vi "QSBEncoder5.vi"() -> ()   [LabVIEW 2010]
uses:
  C:/Develop/USDigital/QSB/Demos/LabView/QSBLabView2010/USDQSB.dll
  Develop/USDigital/QSB/Demos/LabView/QSBLabView2010/USDQSB.dll
  C:/projects/SIMIS/USDigital/QSBLabView2009/USDQSB.dll
  projects/SIMIS/USDigital/QSBLabView2009/USDQSB.dll
panel:
  in  "Detect Crimp":bool
  out "Waiting For Crimp":bool
  out "Signed Count":i32=1
  out "CrimpTime":u32
  out "CrimpStart":u32
  out "Sampling":bool
  in  "stop":bool
  out "Stopped":bool
  out "Encoder Position":dbl[](array[numeric])=[1.0, 1.0, 1.0, 1.0, 1.0, 1.0, 1.0, 1.0, 1.0, 1.0, 1.0, 1.0, 1.0, 1.0, 1.0, 1.0, 1.0, 1.0, 1.0, 1.0, 1.0, 1.0, 1.0, 1.0, 1.0, 1.0, 1.0, 1.0, 1.0, 1.0, 1.0, 1.0, 1.0, 1.0, 1.0, 1.0, 1.0, 1.0, 1.0, 1.0, 1.0, 1.0, 1.0, 1.0, 1.0, 1.0, 1.0, 1.0, 1.0, 1.0, 1.0, 1.0, 1.0, 1.0, 1.0, 1.0, 1.0, 1.0, 1.0, 1.0, 1.0, 1.0, 1.0, 1.0, 1.0, 1.0, 1.0, 1.0, 1.0, 1.0, 1.0, 1.0, 1.0, 1.0, 1.0, 1.0, 1.0, 1.0, 1.0, 1.0, 1.0, 1.0, 1.0, 1.0, 1.0, 1.0, 1.0, 1.0, 1.0, 1.0, 1.0, 1.0, 1.0, 1.0, 1.0, 1.0, 1.0, 1.0, 1.0, 1.0, 1.0, 1.0, 1.0, 1.0, 1.0, 1.0, 1.0, 1.0, 1.0, 1.0, 1.0, 1.0, 1.0, 1.0, 1.0, 1.0, 1.0, 1.0, 1.0, 1.0, 1.0, 1.0, 1.0, 1.0, 1.0, 1.0, 1.0, 1.0, 1.0, 1.0, 1.0, 1.0, 1.0, 1.0, 1.0, 1.0, 1.0, 1.0, 1.0, 1.0, 1.0, 1.0, 1.0, 1.0, 1.0, 1.0, 1.0, 1.0, 1.0, 1.0, 1.0, 1.0, 1.0, 1.0, 1.0, 1.0, 1.0, 1.0, 1.0, 1.0, 1.0, 1.0, 1.0, 1.0, 1.0, 1.0, 1.0, 1.0, 1.0, 1.0, 1.0, 1.0, 1.0, 1.0, 1.0, 1.0, 1.0, 1.0, 1.0, 1.0, 1.0, 1.0, 1.0, 1.0, 0.0, 0.0, 0.0, 0.0, 0.0, 0.0, 0.0, 0.0, 0.0, 0.0, 0.0, 0.0, 0.0, 0.0, 0.0, 0.0, 0.0, 0.0, 0.0, 0.0, 0.0, 0.0, 0.0, 0.0, 0.0, 0.0, 0.0, 0.0, 0.0, 0.0, 0.0, 0.0, 0.0, 0.0, 0.0, 0.0, 0.0, 0.0, 0.0, 0.0, 0.0, 0.0, 0.0, 0.0, 0.0, 0.0, 0.0, 0.0, 0.0, 0.0, 0.0, 0.0, 0.0, 0.0, 0.0, 0.0, 0.0, 0.0, 0.0, 0.0, 0.0, 0.0, 0.0, 0.0, 0.0, 0.0, 0.0, 0.0, 0.0, 0.0, 0.0, 0.0, 0.0, 0.0, 0.0, 0.0, 0.0, 0.0, 0.0, 0.0, 0.0, 0.0, 0.0, 0.0, 0.0, 0.0, 0.0, 0.0, 0.0, 0.0, 0.0, 0.0, 0.0, 0.0, 0.0, 0.0, 0.0, 0.0, 0.0, 0.0, 0.0, 0.0, 0.0, 0.0, 0.0, 0.0, 0.0, 0.0, 0.0, 0.0, 0.0, 0.0, 1.0, 1.0, 1.0, 1.0, 1.0, 1.0, 1.0, 1.0, 1.0, 1.0, 1.0, 1.0, 1.0, 1.0, 1.0, 1.0, 1.0, 1.0, 1.0, 1.0, 1.0, 1.0, 1.0, 1.0, 1.0, 1.0, 1.0, 1.0, 1.0, 1.0, 1.0, 1.0, 1.0, 1.0, 1.0, 1.0, 1.0, 1.0, 1.0, 1.0, 1.0, 1.0, 1.0, 1.0, 1.0, 1.0, 1.0, 1.0, 1.0, 1.0, 1.0, 1.0, 1.0, 1.0, 1.0, 1.0, 1.0, 1.0, 1.0, 1.0, 1.0, 1.0, 1.0, 1.0, 1.0, 1.0, 1.0, 1.0, 1.0, 1.0, 1.0, 1.0, 1.0, 1.0, 1.0, 1.0, 1.0, 1.0, 1.0, 1.0, 1.0, 1.0, 1.0, 1.0, 1.0, 1.0, 1.0, 1.0, 1.0, 1.0, 1.0, 1.0, 1.0, 1.0, 1.0, 1.0, 1.0, 1.0, 1.0, 1.0, 1.0, 1.0, 1.0, 1.0, 1.0, 1.0, 1.0, 1.0, 1.0, 1.0, 1.0, 1.0, 1.0, 1.0, 1.0, 1.0, 1.0, 1.0, 1.0, 1.0, 1.0, 1.0, 1.0, 1.0, 1.0, 1.0, 1.0, 1.0, 1.0, 1.0, 1.0, 1.0, 1.0, 1.0, 1.0, 1.0, 1.0, 1.0, 1.0, 1.0, 1.0, 1.0, 1.0, 1.0, 1.0, 1.0, 1.0, 1.0, 1.0, 1.0, 1.0, 1.0, 1.0, 1.0, 1.0, 1.0, 1.0, 1.0, 1.0, 1.0, 1.0, 1.0, 1.0, 1.0, 1.0, 1.0, 1.0, 1.0, 1.0, 1.0, 1.0, 1.0, 1.0, 1.0, 1.0, 1.0, 1.0, 1.0, 1.0, 1.0, 1.0, 1.0, 1.0, 1.0, 1.0, 1.0, 1.0, 1.0, 1.0, 1.0, 1.0, 1.0, 1.0, 1.0, 1.0, 1.0, 1.0, 1.0, 1.0, 1.0, 1.0, 1.0, 1.0, 1.0] format="%.2f"
  out "waveform output (graph)":waveform(dbl)(graph)
  in  "Range":dbl=40000.0
  out "Current Position":dbl=1.0
  out "Encoder Count":i32(slide)=1 scale=-30000.0..40000.0
  out "Minimum (msec)":u32=4294967295
  out "Maximum (msec)":u32
  out "Numeric":i32
  out "Connected":bool
  in  "Port Name i.e. COM3":string="COM3"
  out "Connection Status":string="Not Connected"
  in  "Connect":bool
  in  "OFF":bool caption="ON"
  out "Invert Direction":bool
  in  "OFF":bool=TRUE caption="ON"
  out "Enable Counter":bool=TRUE
  out "Sign Bit Set":bool=TRUE
  out "Count Increase":bool
  out "Counter Enabled":bool=TRUE
  out "Index":bool=TRUE
  out "Match":bool
  out "Rollunder":bool=TRUE
  out "Rollover":bool=TRUE
  out "Status (hex)":u32=217 format="%x"
  in  "Clear Status":bool caption="Clear"
  in  "OFF":bool caption="ON"
  out "Trigger On Index":bool
  in  "OFF":bool caption="ON"
  in  "OFF":bool caption="ON"
  out "Trigger On Match":bool
  out "Trigger On Rollunder":bool
  in  "OFF":bool caption="ON"
  out "Trigger On Rollover":bool
  in  "Index Configuration":T1(ring)=enum."Reset Counter"
  out "Index Configuration":string="Reset Counter"
  in  "Counter Mode":T2(ring)
  in  "Reset Count":bool caption="Reset"
  out "Resolution":i32=60001
  out "Counter Mode":string="Free Running"
  out "Quadrature Mode":string="X4"
  in  "Quadrature Mode":enum16{"Clock and Direction", "X1", "X2", "X4"}(ring)=enum."X4"
  in  "Apply":bool
  out "error out":errorcluster
  in  "Input Resolution":i32=60001 max=131071 step=100
  in  "error in (no error)":errorcluster
  # "Encoder Configuration"
  # "Encoder Status"
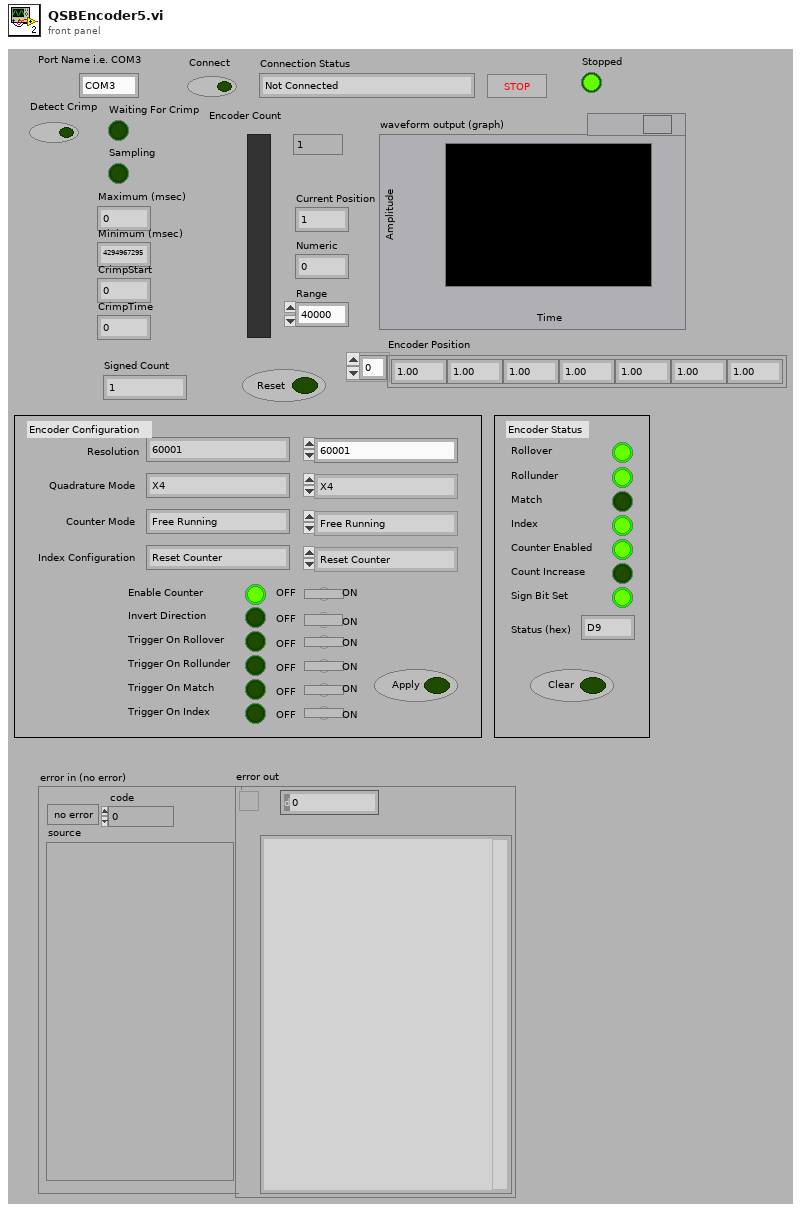
[diagram p1: front panel]
types:
  T1 = enum16{"Disabled", "Preset Counter", "Reset Counter", "Capture Counter"}
  T2 = enum16{"Free Running", "Non-Recycle", "Range Limit", "Modulo-N"}
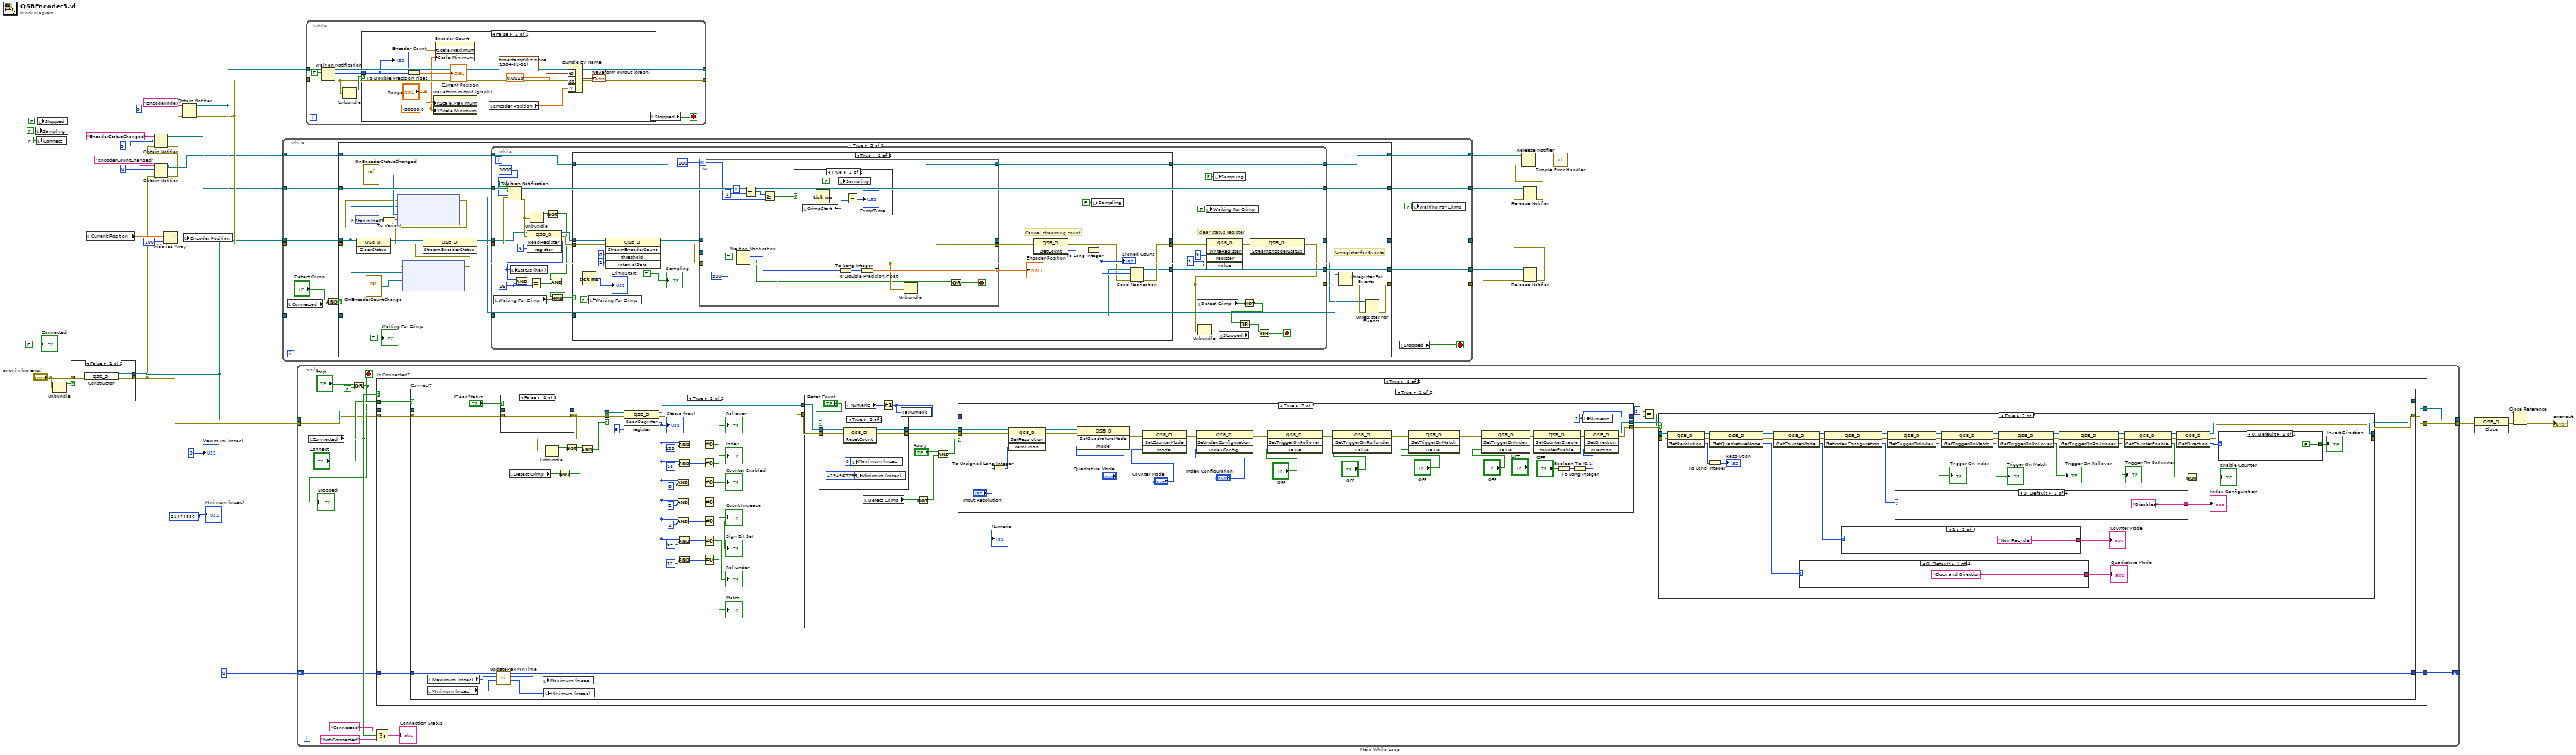
[diagram p0: block diagram]
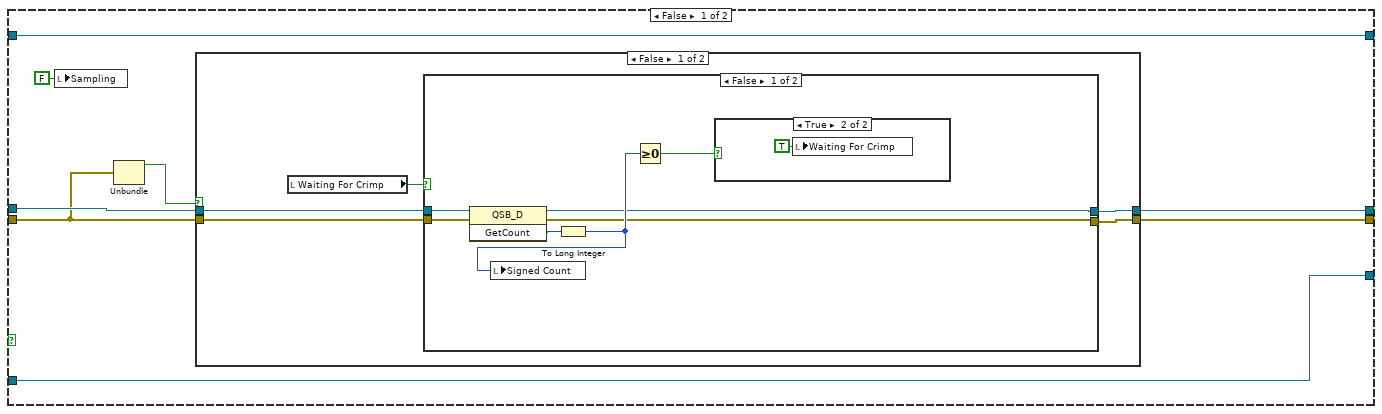
[diagram p4: hidden frame]
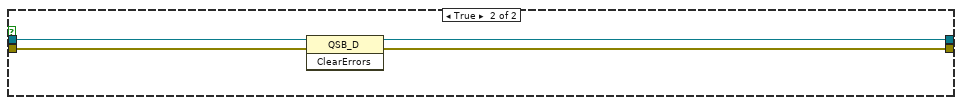
[diagram p7: hidden frame]
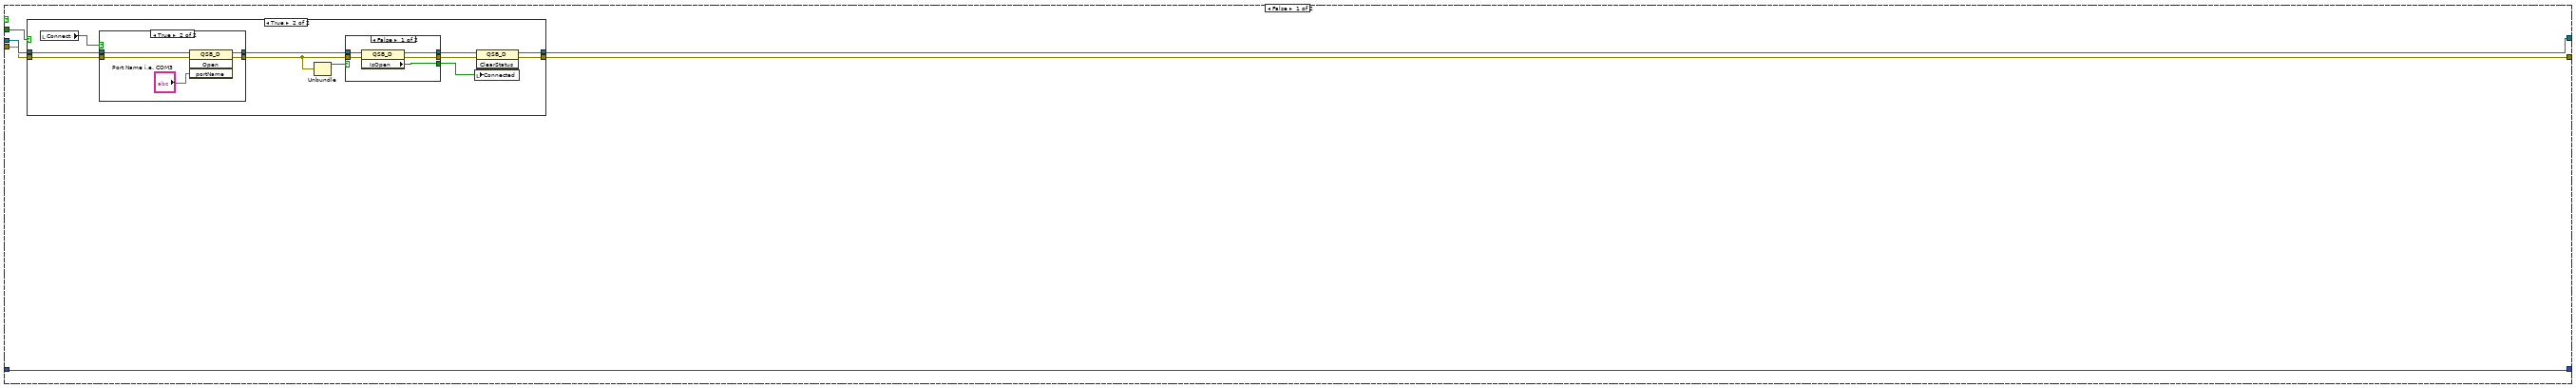
[diagram p9: hidden frame]
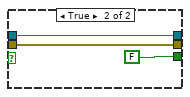
[diagram p11: hidden frame]
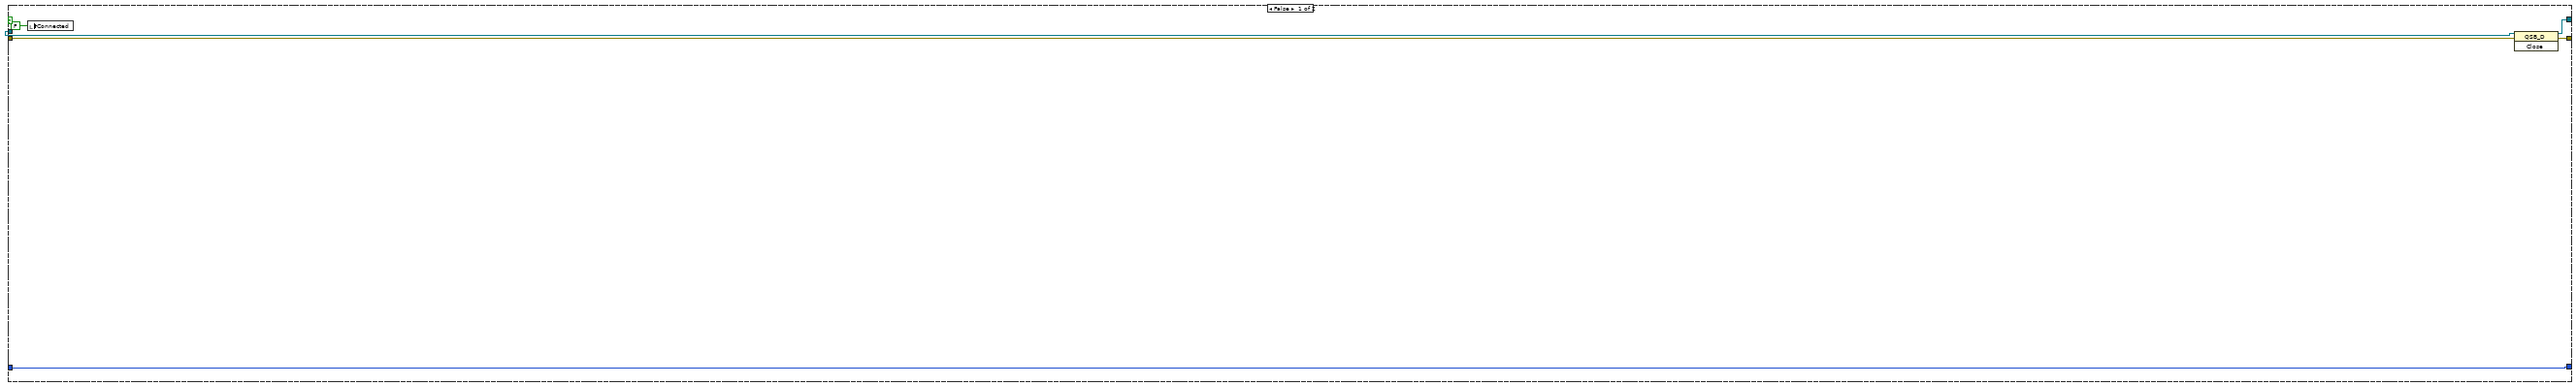
[diagram p13: hidden frame]
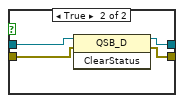
[diagram p15: hidden frame]
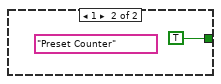
[diagram p18: hidden frame]
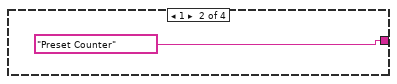
[diagram p19: hidden frame]
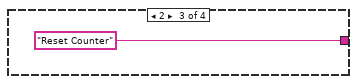
[diagram p20: hidden frame]
diagram:
  n1 = local write "Sampling"(FALSE ("Sampling")) -> ()
  n2 = local write "Connect"(FALSE ("Connect")) -> ()
  n3 = local write "Stopped"(FALSE ("Stopped")) -> ()
  n4 = Unbundle("error in (no error)") -> ("status"=w38:bool)  [unwired: 2 out]
  n5 = case shown="False" w38 {
    tunnel: [w39 refnum<k24> refnum ("new reference")] -> w12
    tunnel: "error in (no error)" -> [w41 w43]
    tunnel: [w40 w43] -> w6
    frame False {
      n6 = constructor class="QSB_D"(error in=w41) -> (reference out=w39:refnum<k24>, error out=w40:errorcluster)  [unwired: 2 in, 1 out]
    }
    frame True {
    }
  }
  n7 = local read "Current Position"() -> (w26:dbl)
  n8 = Obtain Notifier(name (unnamed)="EncoderCountChanged", notification data type=0, error in (no error)=w6) -> (notifier out=w4:refnum<notifier>, error out=w5:errorcluster)  [unwired: 1 in, 1 out]
  n9 = Obtain Notifier(name (unnamed)="EncoderStatusChanged", notification data type=u32 0, error in (no error)=w5) -> (notifier out=w15:refnum<notifier>, error out=w9:errorcluster)  [unwired: 1 in, 1 out]
  n10 = Initialize Array(w26, 100 ("dimension size")) -> (w10:dbl[])
  n11 = Obtain Notifier(name (unnamed)="EncoderIndex", notification data type=0, error in (no error)=w9) -> (notifier out=w24:refnum<notifier>, error out=w23:errorcluster)  [unwired: 1 in, 1 out]
  n12 = local write "Encoder Position"(w10) -> ()
  n13 = while {
    tunnel: w12 -> [w54]
    tunnel: w23 -> [w53]
    tunnel: w24 -> [w58]
    tunnel: [w57] -> w28
    tunnel: [w56] -> w11
    tunnel: w15 -> [w49]
    tunnel: [w47] -> w14
    tunnel: [w46] -> _
    tunnel: w4 -> [w45]
    tunnel: [w44] -> w1
    stop <- w55 stop-if-true
    n14 = local read "Connected"() -> (w51:bool)
    n15 = And(x="Detect Crimp", y=w51) -> (x .and. y?=w52:bool)
    n16 = case shown="True" w52 {
      tunnel: w54 -> [w60 w70]
      tunnel: w53 -> [w63 w76]
      tunnel: w58 -> [w62 w88]
      tunnel: [w62 w87] -> w57
      tunnel: [w63 w66] -> w56
      tunnel: w49 -> [w61 w85]
      tunnel: [w61 w84] -> w47
      tunnel: [w60 w74] -> w46
      tunnel: w45 -> [w59 w73]
      tunnel: [w59 w72] -> w44
      frame False {
      }
      frame True {
        # "Unregister for Events"
        n17 = control-ref of="Status (hex)"() -> (w82:refnum<vi>)
        n18 = invoke class="QSB_D" method="ClearStatus"(reference=w70, error in=w76) -> (reference out=w77:refnum<k24>, error out=w75:errorcluster)  [unwired: 1 in, 1 out]
        n19 = vi-ref <userlib>:"OnEncoderStatusChanged.vi"() -> ("vi reference"=w79:refnum<vi>)
        n20 = vi-ref <userlib>:"OnEncoderCountChange.vi"() -> ("vi reference"=w71:refnum<vi>)
        n21 = To Variant(anything=w82) -> (Variant=w83:variant)
        n22 = node(w75, w70, w79, w83) -> (w65:refnum<k27>, w69:errorcluster)  [unwired: 1 in]
        n23 = node(w69, w70, w71) -> (w64:refnum<k27>, w68:errorcluster)  [unwired: 2 in]
        n24 = invoke class="QSB_D" method="StreamEncoderStatus"(reference=w77, error in=w68) -> (reference out=w81:refnum<k24>, error out=w80:errorcluster)  [unwired: 1 in, 1 out]
        n25 = while {
          tunnel: w80 -> [w118]
          tunnel: w88 -> [w125]
          tunnel: w81 -> [w105]
          tunnel: [w124] -> w87
          tunnel: [w109] -> w78
          tunnel: w85 -> [w119]
          tunnel: [w113] -> w84
          tunnel: [w108] -> w74
          tunnel: w73 -> [w92]
          tunnel: [w91] -> w72
          stop <- w123 stop-if-true
          w126 = u32 16 ("y")
          # "clear status register"
          n26 = local read "Waiting For Crimp"() -> (w96:bool)
          n27 = Wait on Notification(notifier=w119, ignore previous (F)=TRUE, timeout in ms (-1)=1000, error in (no error)=w118) -> (notifier out=w113:refnum<notifier>, error out=w107:errorcluster)  [unwired: 2 out]
          n28 = invoke class="QSB_D" method="ReadRegister"(reference=w105, error in=w107, "register"=u8 6) -> (reference out=w104:refnum<k24>, error out=w106:errorcluster, "ReadRegister"=w94:u32)  [unwired: 1 in, 1 out]
          n29 = local write "Status (hex)"(w94) -> ()
          n30 = And(x=w94, y=w126) -> (x .and. y?=w127:u32)
          n31 = Equal?(x=w127, y=w126) -> (x = y?=w116:bool)
          n32 = Unbundle(w107) -> ("status"=w117:bool)  [unwired: 2 out]
          n33 = Not(x=w117) -> (.not. x?=w95:bool)
          n34 = And(x=w95, y=w116) -> (x .and. y?=w111:bool)
          n35 = And(x=w111, y=w96) -> (x .and. y?=w110:bool)
          n36 = case shown="True" w110 {
            tunnel: w106 -> [w130 w156]
            tunnel: w125 -> [w135 w173]
            tunnel: [w135 w175] -> w124
            tunnel: [w131 w176] -> w99
            tunnel: w104 -> [w133 w163]
            tunnel: [w132 w161] -> w100
            tunnel: w92 -> [w128 w157]
            tunnel: [w128 w159] -> w91
            frame False {
              n37 = local write "Sampling"(FALSE ("Sampling")) -> ()
              n38 = Unbundle(w130) -> ("status"=w129:bool)  [unwired: 2 out]
              n39 = case shown="False" w129 {
                tunnel: w133 -> [w139 w154]
                tunnel: [w138 w152] -> w132
                tunnel: w130 -> [w137 w153]
                tunnel: [w136 w151] -> w131
                frame False {
                  n40 = local read "Waiting For Crimp"() -> (w140:bool)
                  n41 = case shown="False" w140 {
                    tunnel: w139 -> [w147 w150]
                    tunnel: [w142 w150] -> w138
                    tunnel: w137 -> [w146 w149]
                    tunnel: [w141 w149] -> w136
                    frame False {
                      n42 = invoke class="QSB_D" method="GetCount"(reference=w147, error in=w146) -> (reference out=w142:refnum<k24>, error out=w141:errorcluster, "GetCount"=w145:u32)  [unwired: 1 in]
                      n43 = To Long Integer(number=w145) -> (32bit integer=w144:i32)
                      n44 = local write "Signed Count"(w144) -> ()
                      n45 = Greater Or Equal To 0?(x=w144) -> (x >= 0?=w143:bool)
                      n46 = case shown="True" w143 {
                        frame False {
                        }
                        frame True {
                          n47 = local write "Waiting For Crimp"(TRUE ("Waiting For Crimp")) -> ()
                        }
                      }
                    }
                    frame True {
                    }
                  }
                }
                frame True {
                  n48 = invoke class="QSB_D" method="ClearErrors"(reference=w154, error in=w153) -> (reference out=w152:refnum<k24>, error out=w151:errorcluster)  [unwired: 1 in, 1 out]
                }
              }
            }
            frame True {
              # "Cancel streaming count"
              n49 = Tick Count (ms)() -> (millisecond timer value=→"CrimpStart":u32)
              n50 = local write "Waiting For Crimp"(FALSE ("Waiting For Crimp")) -> ()
              n51 = invoke class="QSB_D" method="StreamEncoderCount"(reference=w163, error in=w156, "threshold"=u32 0, "intervalRate"=u32 1) -> (reference out=w165:refnum<k24>, error out=w167:errorcluster)  [unwired: 1 in, 3 out]
              n52 = for {
                N: 100 -> [w190]
                tunnel: [w194] -> w170 mode=indexing
                tunnel: [w184] -> w158
                tunnel: w167 -> [w185]
                tunnel: w165 -> [w186]
                tunnel: [w186] -> w162
                tunnel: w157 -> [w188]
                tunnel: [w187] -> w159
                i -> [w189]
                stop <- w179 stop-if-true
                n53 = Wait on Notification(notifier=w188, ignore previous (F)=TRUE, timeout in ms (-1)=500, error in (no error)=w185) -> (notifier out=w187:refnum<notifier>, notification=w183:i32, timed out?=w178:bool, error out=w184:errorcluster)
                n54 = Add(x=w189, y=1) -> (x+y=w191:i32)
                n55 = Greater Or Equal?(x=w191, y=w190) -> (x >= y?=w192:bool)
                n56 = case shown="True" w192 {
                  frame False {
                  }
                  frame True {
                    n57 = local read "CrimpStart"() -> (w199:u32)
                    n58 = Tick Count (ms)() -> (millisecond timer value=w198:u32)
                    n59 = local write "Sampling"(FALSE ("Sampling")) -> ()
                    n60 = Subtract(x=w198, y=w199) -> (x-y=→"CrimpTime":u32)
                  }
                }
                n61 = To Long Integer(number=w183) -> (32bit integer=w195:i32)
                n62 = To Double Precision Float(number=w195) -> (double precision float=w194:dbl)
                n63 = Unbundle(w184) -> ("status"=w180:bool)  [unwired: 2 out]
                n64 = Or(x=w178, y=w180) -> (x .or. y?=w179:bool)
              }
              "Encoder Position" <- w170
              n65 = invoke class="QSB_D" method="GetCount"(reference=w162, error in=w158) -> (reference out=w161:refnum<k24>, error out=w155:errorcluster, "GetCount"=w160:u32)  [unwired: 1 in]
              n66 = To Long Integer(number=w160) -> (32bit integer=w174:i32)
              "Signed Count" <- w174
              n67 = local write "Sampling"(FALSE ("Sampling")) -> ()
              n68 = Send Notification(notification=w174, notifier=w173, error in (no error)=w155) -> (notifier out=w175:refnum<notifier>, error out=w176:errorcluster)
              "Sampling" <- TRUE ("Sampling")
            }
          }
          n69 = local read "Detect Crimp"() -> (w115:bool)
          n70 = local write "Waiting For Crimp"(TRUE ("Waiting For Crimp")) -> ()
          n71 = invoke class="QSB_D" method="WriteRegister"(reference=w100, error in=w99, "register"=u8 9, "value"=u32 3) -> (reference out=w98:refnum<k24>, error out=w97:errorcluster)  [unwired: 1 in, 3 out]
          n72 = local write "Sampling"(FALSE ("Sampling")) -> ()
          n73 = local read "Stopped"() -> (w120:bool)
          n74 = Not(x=w115) -> (.not. x?=w90:bool)
          n75 = invoke class="QSB_D" method="StreamEncoderStatus"(reference=w98, error in=w97) -> (reference out=w108:refnum<k24>, error out=w109:errorcluster)  [unwired: 1 in, 1 out]
          n76 = Unbundle(w109) -> ("status"=w121:bool)  [unwired: 2 out]
          n77 = Or(x=w90, y=w121) -> (x .or. y?=w122:bool)
          n78 = Or(x=w122, y=w120) -> (x .or. y?=w123:bool)
        }
        n79 = Unregister For Events(event registration refnum=w65, error in=w78) -> (error out=w67:errorcluster)
        n80 = Unregister For Events(event registration refnum=w64, error in=w67) -> (error out=w66:errorcluster)
        "Waiting For Crimp" <- TRUE ("Waiting For Crimp")
      }
    }
    n81 = local read "Stopped"() -> (w55:bool)
    n82 = local write "Waiting For Crimp"(FALSE ("Waiting for Crimp")) -> ()
  }
  n83 = while "Main While Loop" {
    tunnel: [w213] -> w33
    tunnel: [w212] -> w32
    tunnel: w12 -> [w206]
    tunnel: w6 -> [w205]
    shift-right: [w202] -> _
    shift-left: u32 0 -> [w203]
    stop <- w200 stop-if-true
    n84 = local read "Connected"() -> (w209:bool)
    n85 = Or(x="stop", y=FALSE) -> (x .or. y?=w200:bool)
    "Stopped" <- w200
    n86 = Select(t="Connected", s=w209, f="Not Connected") -> (s? t:f=→"Connection Status":string)
    n87 = case "Is Connected?" shown="True" w209 {
      tunnel: [w216 w254] -> w213
      tunnel: [w215 w253] -> w212
      tunnel: "Connect" -> [w219 w252]
      tunnel: w206 -> [w218 w250]
      tunnel: w205 -> [w217 w251]
      tunnel: w203 -> [w214 w249]
      tunnel: [w214 w248] -> w202
      frame False {
        n88 = case shown="True" w219 {
          tunnel: w218 -> [w220 w229]
          tunnel: w217 -> [w221 w228]
          tunnel: [w221 w223] -> w215
          tunnel: [w220 w222] -> w216
          frame False {
          }
          frame True {
            n89 = local read "Connect"() -> (w226:bool)
            n90 = case shown="True" w226 {
              tunnel: [w242 w247] -> w231
              tunnel: [w241 w246] -> w230
              tunnel: w229 -> [w242 w244]
              tunnel: w228 -> [w241 w243]
              frame False {
              }
              frame True {
                n91 = invoke on="Invoke Node" class="QSB_D" method="Open"(reference=w244, error in=w243, "portName"="Port Name i.e. COM3") -> (reference out=w247:refnum<k24>, error out=w246:errorcluster)  [unwired: 1 in, 2 out]
              }
            }
            n92 = Unbundle(w230) -> ("status"=w232:bool)  [unwired: 2 out]
            n93 = case shown="False" w232 {
              tunnel: [w237 w239] -> w224
              tunnel: [w236 w240] -> w225
              tunnel: w231 -> [w234 w239]
              tunnel: w230 -> [w235 w240]
              tunnel: [w233 FALSE] -> w227
              frame False {
                n94 = property class="QSB_D"(reference=w234, error in=w235) -> (reference out=w237:refnum<k24>, error out=w236:errorcluster, "IsOpen"=w233:bool)
              }
              frame True {
              }
            }
            n95 = local write "Connected"(w227) -> ()
            n96 = invoke class="QSB_D" method="ClearStatus"(reference=w224, error in=w225) -> (reference out=w222:refnum<k24>, error out=w223:errorcluster)  [unwired: 1 in, 1 out]
          }
        }
      }
      frame True {
        n97 = case "Connect?" shown="True" w252 {
          tunnel: [w257 w292] -> w254
          tunnel: [w258 w291] -> w253
          tunnel: w251 -> [w260 w277]
          tunnel: w250 -> [w259 w276]
          tunnel: w249 -> [w255 w272]
          tunnel: [w255 w271] -> w248
          frame False {
            n98 = local write "Connected"(FALSE) -> ()
            n99 = invoke class="QSB_D" method="Close"(reference=w259, error in=w260) -> (reference out=w257:refnum<k24>, error out=w258:errorcluster)  [unwired: 1 in, 1 out]
          }
          frame True {
            n100 = local read "Minimum (msec)"() -> (w269:u32)
            n101 = local read "Maximum (msec)"() -> (w270:u32)
            n102 = call <userlib>:"UpdateMaxMinTime.vi"("Minimum (msec)"=w269, "Maximum (msec)"=w270, "LastTime (msec)"=w272) -> ("MinimumOut (msec)"=w267:u32, "MaximumOut (msec)"=w268:u32, "LastTimeOut (msec)"=w271:u32)  [unwired: 6 in]
            n103 = case shown="False" "Clear Status" {
              tunnel: [w303 w307] -> w287
              tunnel: [w304 w305] -> w286
              tunnel: w276 -> [w303 w308]
              tunnel: w277 -> [w304 w306]
              frame False {
              }
              frame True {
                n104 = invoke class="QSB_D" method="ClearStatus"(reference=w308, error in=w306) -> (reference out=w307:refnum<k24>, error out=w305:errorcluster)  [unwired: 1 in, 1 out]
              }
            }
            n105 = local read "Detect Crimp"() -> (w275:bool)
            n106 = local write "Maximum (msec)"(w268) -> ()
            n107 = local write "Minimum (msec)"(w267) -> ()
            n108 = Unbundle(w286) -> ("status"=w265:bool)  [unwired: 2 out]
            n109 = Not(x=w275) -> (.not. x?=w274:bool)
            n110 = Not(x=w265) -> (.not. x?=w266:bool)
            n111 = And(x=w266, y=w274) -> (x .and. y?=w273:bool)
            n112 = case shown="True" w273 {
              tunnel: w286 -> [w310 w337]
              tunnel: w287 -> [w309 w336]
              tunnel: [w309 w335] -> w284
              tunnel: [w310 w333] -> w285
              frame False {
              }
              frame True {
                n113 = invoke on="Invoke Node" class="QSB_D" method="ReadRegister"(reference=w336, error in=w337, "register"=6) -> (reference out=w335:refnum<k24>, error out=w333:errorcluster, "ReadRegister"=w311:u32)  [unwired: 1 in, 1 out]
                "Status (hex)" <- w311
                n114 = And(x=w311, y=8) -> (x .and. y?=w319:u32)
                n115 = And(x=w311, y=2) -> (x .and. y?=w316:u32)
                n116 = And(x=w311, y=1) -> (x .and. y?=w313:u32)
                n117 = And(x=w311, y=128) -> (x .and. y?=w331:u32)
                n118 = And(x=w311, y=16) -> (x .and. y?=w322:u32)
                n119 = And(x=w311, y=64) -> (x .and. y?=w328:u32)
                n120 = And(x=w311, y=32) -> (x .and. y?=w325:u32)
                n121 = Not Equal To 0?(x=w331) -> (x != 0?=→"Rollover":bool)
                n122 = Not Equal To 0?(x=w322) -> (x != 0?=→"Index":bool)
                n123 = Not Equal To 0?(x=w319) -> (x != 0?=→"Counter Enabled":bool)
                n124 = Not Equal To 0?(x=w316) -> (x != 0?=→"Count Increase":bool)
                n125 = Not Equal To 0?(x=w313) -> (x != 0?=→"Sign Bit Set":bool)
                n126 = Not Equal To 0?(x=w328) -> (x != 0?=→"Rollunder":bool)
                n127 = Not Equal To 0?(x=w325) -> (x != 0?=→"Match":bool)
              }
            }
            n128 = case shown="True" "Reset Count" {
              tunnel: w285 -> [w295 w302]
              tunnel: w284 -> [w296 w301]
              tunnel: [w296 w300] -> w283
              tunnel: [w295 w299] -> w282
              frame False {
              }
              frame True {
                n129 = invoke class="QSB_D" method="ResetCount"(reference=w301, error in=w302) -> (reference out=w300:refnum<k24>, error out=w299:errorcluster)  [unwired: 1 in, 1 out]
                n130 = local write "Maximum (msec)"(u32 0 ("Maximum (msec)")) -> ()
                n131 = local write "Minimum (msec)"(u32 4294967295 ("Minimum (msec)")) -> ()
              }
            }
            n132 = local read "Numeric"() -> (w290:i32)
            n133 = local read "Detect Crimp"() -> (w262:bool)
            n134 = Increment(x=w290) -> (x+1=w289:i32)
            n135 = local write "Numeric"(w289) -> ()
            n136 = Not(x=w262) -> (.not. x?=w264:bool)
            n137 = And(x="Apply", y=w264) -> (x .and. y?=w263:bool)
            n138 = case shown="True" w263 {
              tunnel: w282 -> [w394 w400]
              tunnel: w283 -> [w393 w399]
              tunnel: [w393 w403] -> w293
              tunnel: [w394 w402] -> w294
              tunnel: w289 -> [w392 _]
              tunnel: [w392 w426] -> w279
              frame False {
              }
              frame True {
                w426 = 1
                n139 = To Unsigned Long Integer(number="Input Resolution") -> (unsigned 32bit integer=w404:u32)
                n140 = invoke class="QSB_D" method="SetResolution"(reference=w399, error in=w400, "resolution"=w404) -> (reference out=w397:refnum<k24>, error out=w398:errorcluster)  [unwired: 1 in, 2 out]
                n141 = invoke class="QSB_D" method="SetQuadratureMode"(reference=w397, error in=w398, "mode"="Quadrature Mode") -> (reference out=w430:refnum<k24>, error out=w429:errorcluster)  [unwired: 1 in, 2 out]
                n142 = invoke class="QSB_D" method="SetCounterMode"(reference=w430, error in=w429, "mode"="Counter Mode") -> (reference out=w428:refnum<k24>, error out=w427:errorcluster)  [unwired: 1 in, 2 out]
                n143 = invoke class="QSB_D" method="SetIndexConfiguration"(reference=w428, error in=w427, "indexConfig"="Index Configuration") -> (reference out=w422:refnum<k24>, error out=w421:errorcluster)  [unwired: 1 in, 2 out]
                n144 = invoke class="QSB_D" method="SetTriggerOnRollover"(reference=w422, error in=w421, "value"="OFF") -> (reference out=w425:refnum<k24>, error out=w420:errorcluster)  [unwired: 1 in, 2 out]
                n145 = invoke class="QSB_D" method="SetTriggerOnRollunder"(reference=w425, error in=w420, "value"="OFF") -> (reference out=w424:refnum<k24>, error out=w419:errorcluster)  [unwired: 1 in, 2 out]
                n146 = invoke class="QSB_D" method="SetTriggerOnMatch"(reference=w424, error in=w419, "value"="OFF") -> (reference out=w423:refnum<k24>, error out=w418:errorcluster)  [unwired: 1 in, 2 out]
                n147 = invoke class="QSB_D" method="SetTriggerOnIndex"(reference=w423, error in=w418, "value"="OFF") -> (reference out=w408:refnum<k24>, error out=w405:errorcluster)  [unwired: 1 in, 2 out]
                n148 = invoke class="QSB_D" method="SetCounterEnable"(reference=w408, error in=w405, "counterEnable"="OFF") -> (reference out=w407:refnum<k24>, error out=w406:errorcluster)  [unwired: 1 in, 2 out]
                n149 = Boolean To (0,1)(Boolean="OFF") -> (0, 1=w396:i16)
                n150 = To Long Integer(number=w396) -> (32bit integer=w395:i32)
                n151 = local write "Numeric"(w426) -> ()
                n152 = invoke class="QSB_D" method="SetDirection"(reference=w407, error in=w406, "direction"=w395) -> (reference out=w403:refnum<k24>, error out=w402:errorcluster)  [unwired: 1 in, 2 out]
              }
            }
            n153 = Equal?(x=1, y=w279) -> (x = y?=w278:bool)
            n154 = case shown="True" w278 {
              tunnel: w294 -> [w339 w377]
              tunnel: w293 -> [w338 w376]
              tunnel: [w338 w347] -> w292
              tunnel: [w339 w346] -> w291
              frame False {
              }
              frame True {
                n155 = invoke class="QSB_D" method="GetResolution"(reference=w376, error in=w377) -> (reference out=w375:refnum<k24>, error out=w373:errorcluster, "GetResolution"=w341:u32)  [unwired: 1 in]
                n156 = To Long Integer(number=w341) -> (32bit integer=→"Resolution":i32)
                n157 = invoke class="QSB_D" method="GetQuadratureMode"(reference=w375, error in=w373) -> (reference out=w374:refnum<k24>, error out=w372:errorcluster, "GetQuadratureMode"=w370:i32)  [unwired: 1 in]
                n158 = invoke class="QSB_D" method="GetCounterMode"(reference=w374, error in=w372) -> (reference out=w367:refnum<k24>, error out=w366:errorcluster, "GetCounterMode"=w369:i32)  [unwired: 1 in]
                n159 = case shown="0, Default" w370 {
                  tunnel: ["Clock and Direction" "X1" "X2" "X4"] -> w371
                  frame 0, Default {
                  }
                  frame 1 {
                  }
                  frame 2 {
                  }
                  frame 3 {
                  }
                }
                "Quadrature Mode" <- w371
                n160 = invoke class="QSB_D" method="GetIndexConfiguration"(reference=w367, error in=w366) -> (reference out=w363:refnum<k24>, error out=w359:errorcluster, "GetIndexConfiguration"=w365:i32)  [unwired: 1 in]
                n161 = case shown="1" w369 {
                  tunnel: ["Free Running" "Non Recycle" "Range Limit" "Modulo-N"] -> w368
                  frame 0 {
                  }
                  frame 1 {
                  }
                  frame 2 {
                  }
                  frame 3, Default {
                  }
                }
                "Counter Mode" <- w368
                n162 = invoke class="QSB_D" method="GetTriggerOnIndex"(reference=w363, error in=w359) -> (reference out=w362:refnum<k24>, error out=w358:errorcluster, "GetTriggerOnIndex"=→"Trigger On Index":bool)  [unwired: 1 in]
                n163 = case shown="0, Default" w365 {
                  tunnel: ["Disabled" "Preset Counter" "Reset Counter" "Capture Counter"] -> w364
                  frame 0, Default {
                  }
                  frame 1 {
                  }
                  frame 2 {
                  }
                  frame 3 {
                  }
                }
                "Index Configuration" <- w364
                n164 = invoke class="QSB_D" method="GetTriggerOnMatch"(reference=w362, error in=w358) -> (reference out=w361:refnum<k24>, error out=w357:errorcluster, "GetTriggerOnMatch"=→"Trigger On Match":bool)  [unwired: 1 in]
                n165 = invoke class="QSB_D" method="GetTriggerOnRollover"(reference=w361, error in=w357) -> (reference out=w360:refnum<k24>, error out=w356:errorcluster, "GetTriggerOnRollover"=→"Trigger On Rollover":bool)  [unwired: 1 in]
                n166 = invoke class="QSB_D" method="GetTriggerOnRollunder"(reference=w360, error in=w356) -> (reference out=w351:refnum<k24>, error out=w350:errorcluster, "GetTriggerOnRollunder"=→"Trigger On Rollunder":bool)  [unwired: 1 in]
                n167 = invoke class="QSB_D" method="GetCounterEnable"(reference=w351, error in=w350) -> (reference out=w349:refnum<k24>, error out=w348:errorcluster, "GetCounterEnable"=w343:bool)  [unwired: 1 in]
                n168 = invoke class="QSB_D" method="GetDirection"(reference=w349, error in=w348) -> (reference out=w347:refnum<k24>, error out=w346:errorcluster, "GetDirection"=w345:i32)  [unwired: 1 in]
                n169 = Not(x=w343) -> (.not. x?=→"Enable Counter":bool)
                n170 = case shown="0, Default" w345 {
                  tunnel: [FALSE TRUE] -> w344
                  frame 0, Default {
                  }
                  frame 1 {
                    (unwired) "Preset Counter"
                  }
                }
                "Invert Direction" <- w344
              }
            }
          }
        }
      }
    }
  }
  n171 = while {
    tunnel: w24 -> [w438]
    tunnel: w23 -> [w437]
    tunnel: [w433] -> _
    tunnel: [w432] -> _
    stop <- w435 stop-if-true
    n172 = Wait on Notification(notifier=w438, ignore previous (F)=TRUE, error in (no error)=w437) -> (notifier out=w433:refnum<notifier>, notification=w436:i32, error out=w432:errorcluster)  [unwired: 1 in, 1 out]
    n173 = Unbundle(w432) -> ("status"=w434:bool)  [unwired: 2 out]
    n174 = case shown="False" w434 {
      tunnel: w436 -> [w443 _]
      frame False {
        w440 = -30000.0
        n175 = To Double Precision Float(number=w443) -> (double precision float=→"Current Position":dbl)
        n176 = property on="waveform output (graph)" class="WFGraph (strict)"("YScale.Maximum"="Range", "YScale.Minimum"=w440) -> ()  [unwired: 2 in, 2 out]
        n177 = property on="Encoder Count" class="Slide (strict)"("Scale.Maximum"="Range", "Scale.Minimum"=w440) -> ()  [unwired: 2 in, 2 out]
        n178 = local read "Encoder Position"() -> (w439:dbl[])
        n179 = Bundle By Name ("Build Waveform")("t0"=timestamp(0 s since 1904-01-01), "dt"=0.0019, "Y"=w439) -> (→"waveform output (graph)":waveform(dbl))  [unwired: 1 in]
        "Encoder Count" <- w443
      }
      frame True {
      }
    }
    n180 = local read "Stopped"() -> (w435:bool)
  }
  n181 = Release Notifier(notifier=w28, error in (no error)=w11) -> (error out=w13:errorcluster)  [unwired: 1 in, 2 out]
  n182 = Release Notifier(notifier=w14, error in (no error)=w13) -> (error out=w3:errorcluster)  [unwired: 1 in, 2 out]
  n183 = Release Notifier(notifier=w1, error in (no error)=w3) -> (error out=w2:errorcluster)  [unwired: 1 in, 2 out]
  n184 = call <vilib>:"Simple Error Handler.vi"("error in (no error)"=w2) -> ()  [unwired: 4 in, 5 out]
  n185 = invoke class="QSB_D" method="Close"(reference=w33, error in=w32) -> (reference out=w35:refnum<k24>, error out=w36:errorcluster)  [unwired: 1 in, 1 out]
  n186 = Close Reference(reference=w35, error in (no error)=w36) -> (error out=→"error out":errorcluster)
  "Connected" <- FALSE
  "Maximum (msec)" <- u32 0
  "Minimum (msec)" <- u32 2147483647
